vi "DeactivateAnalogCurrentSettingValue.vi"(4 "error in (no error)":errorcluster, 6 "analogInputNumber":u16, 7 "axis in":cluster{"keyHandle":u32, "nodeId":u16}={"keyHandle"=0, "nodeId"=1}) -> (0 "error out":errorcluster, 3 "axis out":cluster{"keyHandle":u32, "nodeId":u16}={"keyHandle"=0, "nodeId"=1})   [LabVIEW 2010]
doc: "<B>DeactivateAnalogCurrentSettingValue</B> disables the selected analog input for analog current setpoint."
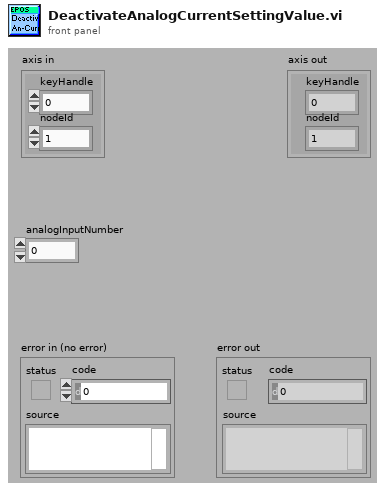
[diagram p1: front panel]
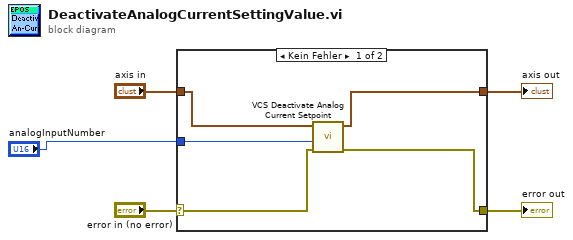
[diagram p0: block diagram]
diagram:
  n1 = case shown="Kein Fehler" "error in (no error)" {
    selector: "error in (no error)" -> [w7 w12]
    tunnel: [w8 w12] -> w4
    tunnel: [w9 w11] -> w3
    tunnel: "axis in" -> [w10 w11]
    tunnel: "analogInputNumber" -> [w6 _]
    frame No Error {
      n2 = call "VCS Deactivate Analog Current Setpoint.vi"("error in (no error)"=w7, "analogInputNumber"=w6, "axis in"=w10) -> ("error out"=w8:errorcluster, "axis out"=w9:cluster{"keyHandle":u32, "nodeId":u16})  [unwired: 7 in]
    }
    frame Error {
    }
  }
  "error out" <- w4
  "axis out" <- w3
